vi "Controller_up.vi"(0 "name 2":string, 5 "port or service name":u16=16389, 7 "connection ID":refnum<k16>, 9 "error in (no error)":errorcluster, 11 "x":dbl[](array[numeric])) -> (4 "*(type *) &x":dbl[](array[numeric]), 6 "error out":errorcluster, 8 "connection ID out":refnum<k16>)   [LabVIEW 2021]
panel:
  out "port":u16
  out "name":string
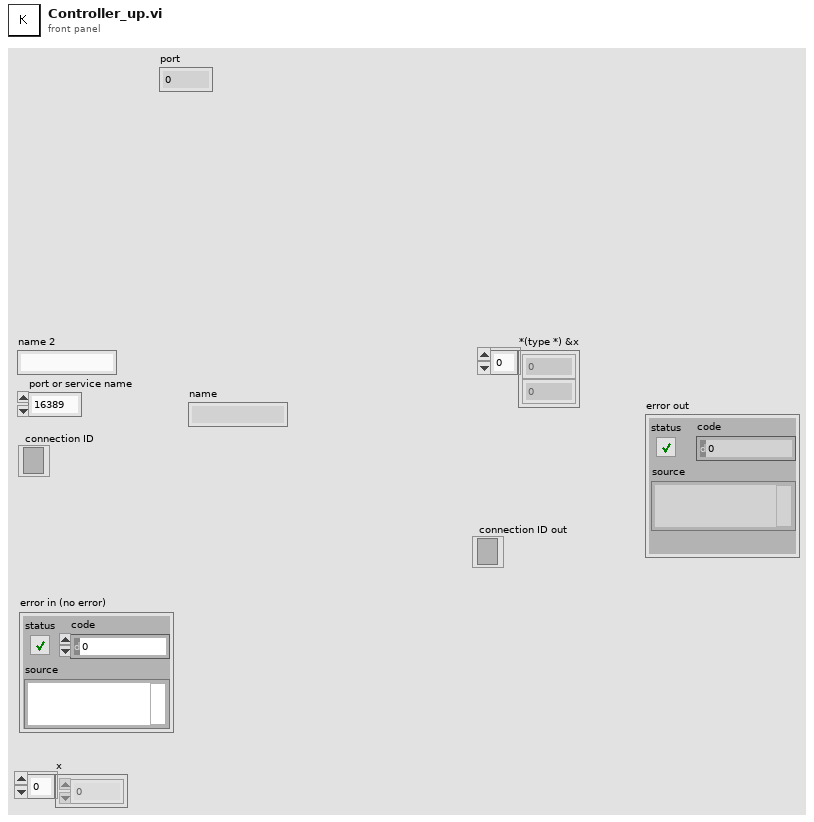
[diagram p1: front panel]
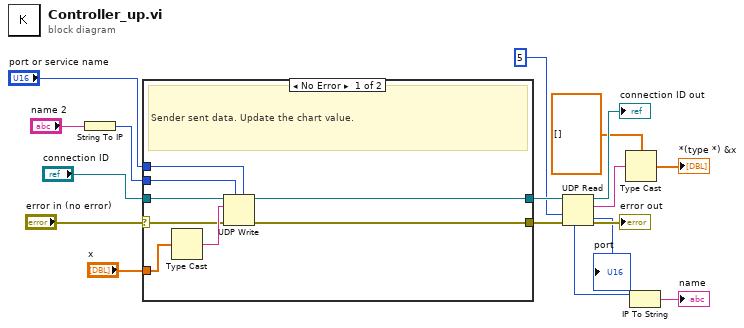
[diagram p0: block diagram]
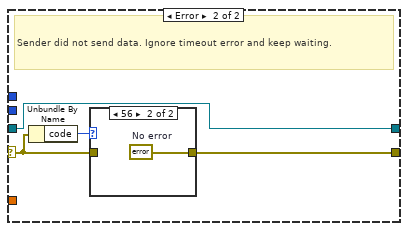
[diagram p2: hidden frame]
diagram:
  n1 = String To IP(1:"name 2") -> (0:w15:u32)
  n2 = case shown="No Error" "error in (no error)" {
    selector: "error in (no error)" -> [w20 w28]
    tunnel: [w19 w27] -> w12
    tunnel: "connection ID" -> [w25 w26]
    tunnel: "port or service name" -> [w24 _]
    tunnel: w15 -> [w23 _]
    tunnel: "x" -> [w21 _]
    tunnel: [w18 w26] -> w11
    frame No Error {
      # "Sender sent data. Update the chart value."
      n3 = Type Cast(x=w21) -> (*(type *) &x=w22:string)  [unwired: 1 in]
      n4 = UDP Write(address=w23, port or service name=w24, connection ID=w25, data in=w22, 8:w20) -> (error out=w19:errorcluster, 3:w18:refnum<k16>)  [unwired: 1 in]
    }
    frame Error {
      # "Sender did not send data. Ignore timeout error and keep waiting."
      n5 = Unbundle By Name(w28) -> ("code"=w29:i32)
      n6 = case shown="56" w29 {
        tunnel: w28 -> [w30 _]
        tunnel: [w30 w31] -> w27
        frame Default {
        }
        frame 56 {
          w31 = errorcluster {"status"=FALSE, "code"=0, "source"=""}  # No error
        }
      }
    }
  }
  n7 = UDP Read(connection ID=w11, timeout ms (25000)=5, 8:w12) -> (data out=w9:string, error out=→"error out":errorcluster, 3:→"connection ID out":refnum<k16>, 4:→"port":u16, 6:w7:u32)  [unwired: 1 out]
  n8 = Type Cast(type=dbl[] [], x=w9) -> (*(type *) &x=→"*(type *) &x":dbl[])
  n9 = IP To String(2:w7) -> (0:→"name":string)  [unwired: 1 in]
